vi "WidgetCenter.vi"(6 "error in":errorcluster, 9 "Control in":refnum<class "Control.lvclass">) -> (0 "error out":errorcluster, 3 "Control out":refnum<class "Control.lvclass">, 4 "Center":T1)   [LabVIEW 2014, in "Raspberry Pi Compatible Compiler for LabVIEW.lvlib" / "Control.lvclass"]
uses:
  Control.lvclass
  <vilib>/Utility/miscctls.llb/LVPositionTypeDef.ctl
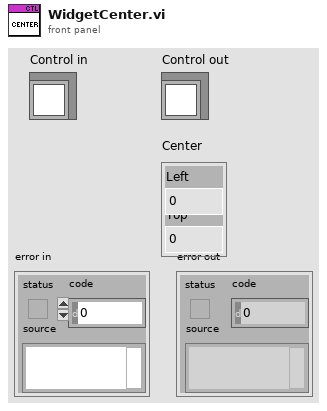
[diagram p1: front panel]
types:
  T1 = typedef "LVPositionTypeDef.ctl" = cluster{"Left":i32, "Top":i32}
  T2 = typedef "LVRectTypeDef.ctl" = cluster{"Left":i16, "Top":i16, "Right":i16, "Bottom":i16}
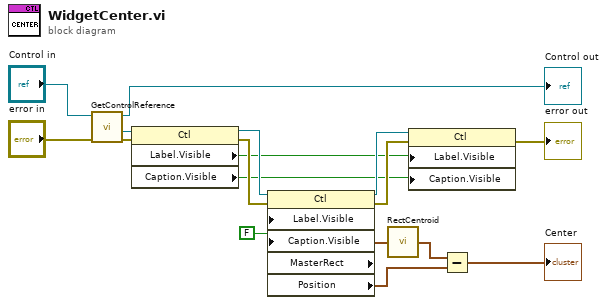
[diagram p0: block diagram]
diagram:
  w11 = FALSE ("Label.Visible")
  n1 = call "GetControlReference.vi"("error in"="error in", "Control in"="Control in") -> ("error out"=w14:errorcluster, "control reference"=w15:refnum<vi>, "Control out"=→"Control out":refnum<class "Control.lvclass">)  [unwired: 7 in]
  n2 = property class="Ctl"(reference=w15, error in=w14) -> (reference out=w12:refnum<vi>, error out=w13:errorcluster, "Label.Visible"=w8:bool, "Caption.Visible"=w7:bool)
  n3 = property class="Ctl"(reference=w12, error in=w13, "Label.Visible"=w11, "Caption.Visible"=w11) -> (reference out=w9:refnum<vi>, error out=w10:errorcluster, "MasterRect"=w4:T2, "Position"=w2:T1)
  n4 = call <vilib>:"RectCentroid.vi"("rect"=w4) -> ("point"=w3:cluster{"x":i16, "y":i16})
  n5 = property class="Ctl"(reference=w9, error in=w10, "Label.Visible"=w8, "Caption.Visible"=w7) -> (error out=→"error out":errorcluster)  [unwired: 1 out]
  n6 = Subtract(x=w3, y=w2) -> (x-y=→"Center":T1)
